vi "Read UIRef.vi"(8 "error in (no error)":errorcluster, 9 "0Arrive/1Finish":i32, 10 "UI Ref":T1, 11 "Station Action in":refnum<class "Station Action.lvclass">) -> (0 "error out":errorcluster, 2 "RefOut":refnum<vi>, 3 "Station Action out":refnum<class "Station Action.lvclass">)   [LabVIEW 2019, in "Station Action.lvclass"]
uses:
  Station Action.lvclass
  Ctrl/Auto Inspection Main UI Ref.ctl
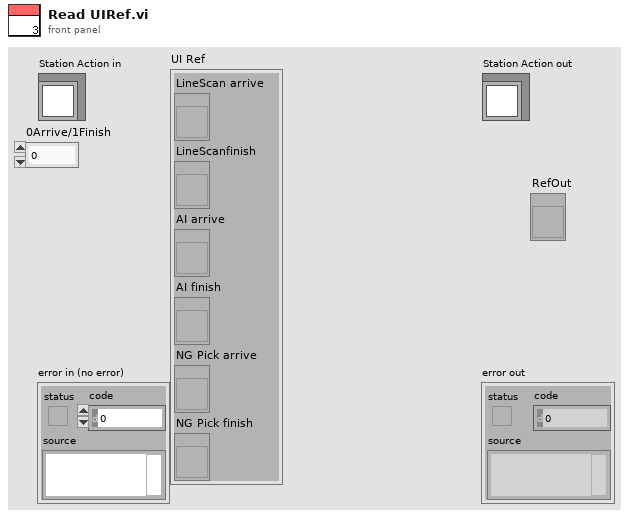
[diagram p1: front panel]
types:
  T1 = typedef "Auto Inspection Main UI Ref.ctl" = cluster{"LineScan arrive":refnum<vi>, "LineScanfinish":refnum<vi>, "AI arrive":refnum<vi>, "AI finish":refnum<vi>, "NG Pick arrive":refnum<vi>, "NG Pick finish":refnum<vi>}
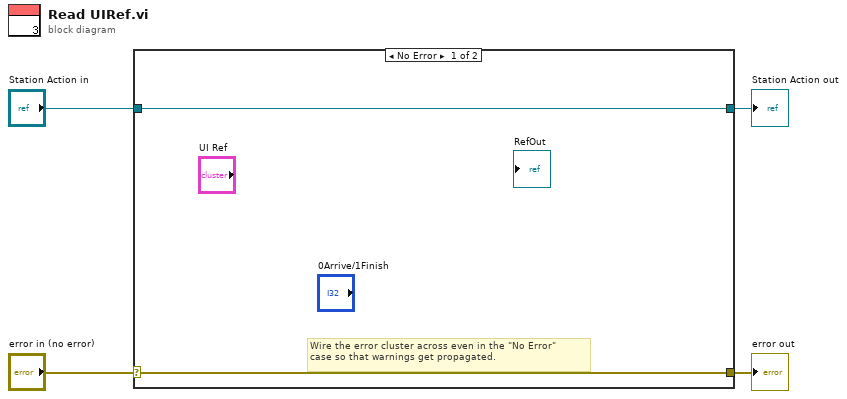
[diagram p0: block diagram]
diagram:
  n1 = case shown="No Error" "error in (no error)" {
    selector: "error in (no error)" -> [w5 w8]
    tunnel: [w5 w8] -> w3
    tunnel: [w6 w7] -> w1
    tunnel: "Station Action in" -> [w6 w7]
    frame No Error {
      # "Wire the error cluster across even in the \"No Error\"\ncase so that warnings get propagated."
    }
    frame Error {
    }
  }
  "error out" <- w3
  "Station Action out" <- w1
